vi "Image_Capture_NI-IMAQdx.vi"(0 "Session In":T2) -> (4 "error out":errorcluster, 6 "Image":T1(plugin-control))   [LabVIEW 2017]
uses:
  <vilib>/userdefined/High Color/IMAQdx.ctl
  <vilib>/vision/driver/NI_Vision_Acquisition_Software.lvlib
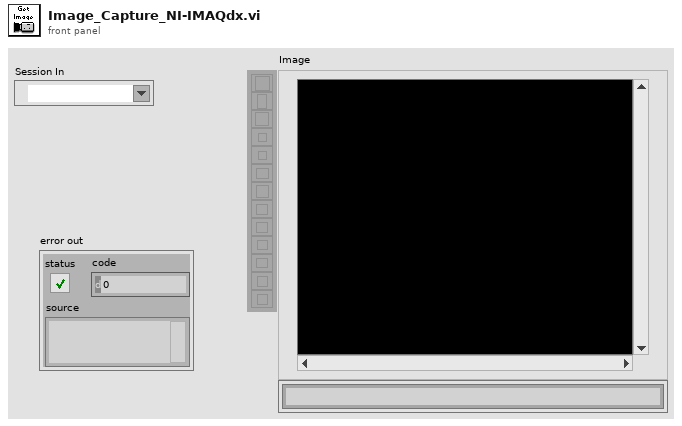
[diagram p1: front panel]
types:
  T1 = typedef "IMAQ Image.ctl" = refnum<image>
  T2 = typedef "IMAQdx.ctl" = refnum<k21>
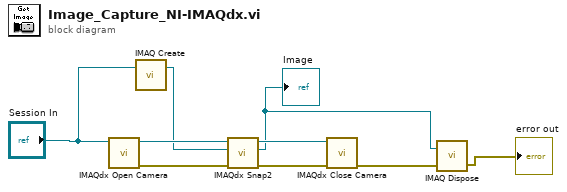
[diagram p0: block diagram]
diagram:
  n1 = call <vilib>:"IMAQdx Open Camera.vi"("Session In"="Session In") -> ("error out"=w4:errorcluster, "Session Out"=w8:T2)  [unwired: 9 in]
  n2 = call "IMAQ Create"("Image Name"="Session In") -> ("New Image"=w7:T1)  [unwired: 4 in, 1 out]
  n3 = call <vilib>:"IMAQdx Snap2.vi"("error in"=w4, "Image In"=w7, "Session In"=w8) -> ("error out"=w3:errorcluster, "Image Out"=w5:T1, "Session Out"=w6:T2)  [unwired: 6 in]
  "Image" <- w5
  n4 = call <vilib>:"IMAQdx Close Camera.vi"("error in"=w3, "Session In"=w6) -> ("error out"=w2:errorcluster)  [unwired: 9 in]
  n5 = call "IMAQ Dispose"("Image"=w5, "error in (no error)"=w2) -> ("error out"=→"error out":errorcluster)  [unwired: 4 in]
